vi "liblisten_retrieve_listen_result_parameter.vi"(8 "error in (no error)":errorcluster, 11 "input":i32) -> (0 "error out":errorcluster, 2 "parameter":string)   [LabVIEW 2015]
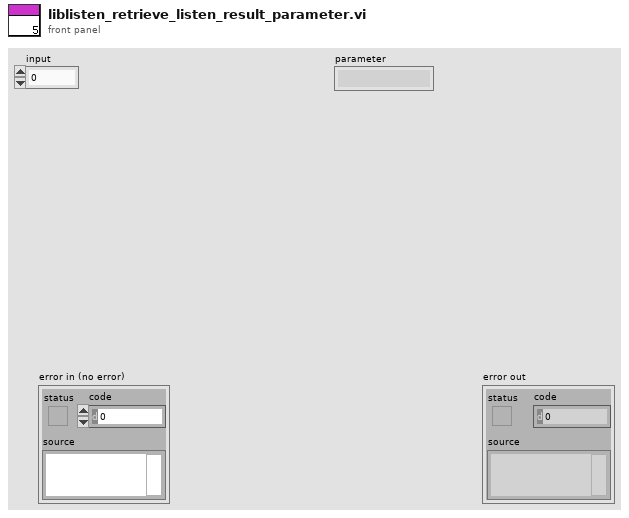
[diagram p1: front panel]
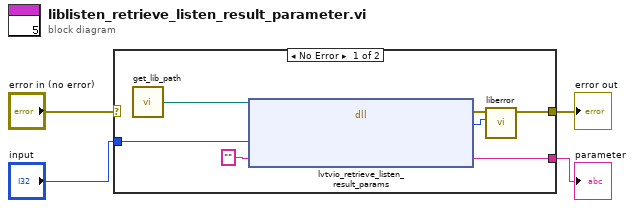
[diagram p0: block diagram]
diagram:
  n1 = case shown="No Error" "error in (no error)" {
    selector: "error in (no error)" -> [_ w12]
    tunnel: [w5 w12] -> w3
    tunnel: [w9 _] -> w2
    tunnel: "input" -> [w8 _]
    frame No Error {
      n2 = call "get_lib_path.vi"() -> ("Path"=w10:path)
      n3 = dll-call lib="S:/thingiverselv/lib/liblvtvio.dll" fn="lvtvio_retrieve_listen_result_params"(path in=w10, "input"=w8, "params"="" ("id")) -> (error out=w6:errorcluster, "return type"=w7:i32, "params"=w9:string)  [unwired: 3 in, 1 out]
      n4 = call "liberror.vi"("tvio errors"=w7, "error in (no error)"=w6) -> ("error out"=w5:errorcluster)  [unwired: 9 in]
    }
    frame Error {
    }
  }
  "error out" <- w3
  "parameter" <- w2
